vi "SW_Prepare_Conditions_Array_for_Saving.vi"(3 "Conditions presets array in":T2 {"Response"."TTL pulse length, ms" min=0.0 max=10000.0 step=10.0 format="%0.0g"; "Specifier(s)"."Validity criteria(s)"."Validity value" min=0.0 step=0.1 format="%.2g"; "Specifier(s)"."Value" step=1.0 format="%#.2g"}) -> (1 "Condition presets prepared for saving out":T1)   [LabVIEW 2018, in "Tracker.lvlib"]
uses:
  Tracker.lvlib
  Controls/CTL_Conditions_Array.ctl
  Controls/CTL_Conditions_Cluster.ctl
  Controls/CTL_Condition_type.ctl
  Controls/CTL_Comparison_type.ctl
  Controls/CTL_Validity_check_criteria.ctl
  Controls/CTL_Condition_response_type.ctl
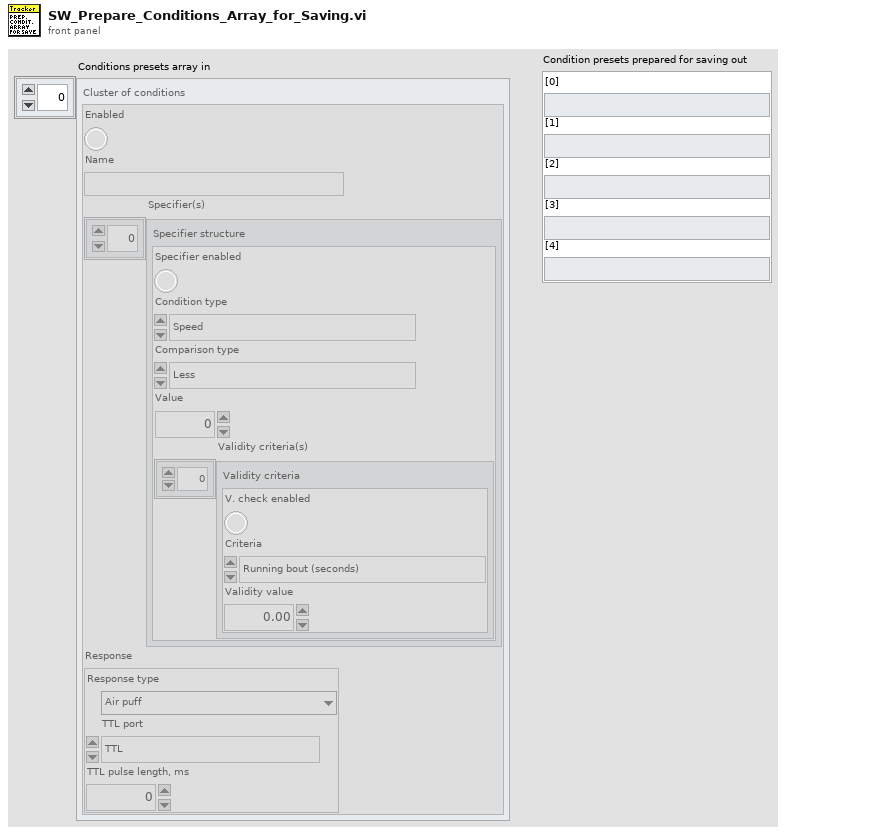
[diagram p1: front panel]
types:
  T1 = cluster{"[0]":string, "[1]":string, "[2]":string, "[3]":string, "[4]":string}
  T2 = typedef "Tracker.lvlib/CTL_Conditions_Array.ctl" = T3[]
  T3 = typedef "Tracker.lvlib/CTL_Conditions_Cluster.ctl" = cluster{"Enabled":bool, "Name":string, "Specifier(s)":cluster{"Specifier enabled":bool, "Condition type":T4, "Comparison type":T5, "Value":dbl, "Validity criteria(s)":cluster{"V. check enabled":bool, "Criteria":T6, "Validity value":dbl}[]}[], "Response":cluster{"Response type":T7, "TTL port":enum16{"TTL"}, "TTL pulse length, ms":dbl}}
  T4 = typedef "Tracker.lvlib/CTL_Condition_type.ctl" = enum16{"Speed", "Zone", "Angle to wall"}
  T5 = typedef "Tracker.lvlib/CTL_Comparison_type.ctl" = enum16{"Less", "Less or Equal", "Equal", "Greater or Equal", "Greater", "Not Equal"}
  T6 = typedef "Tracker.lvlib/CTL_Validity_check_criteria.ctl" = enum16{"Running bout (seconds)", "Running bout (meters)"}
  T7 = typedef "Tracker.lvlib/CTL_Condition_response_type.ctl" = enum16{"None", "Air puff", "Liquid reward"}
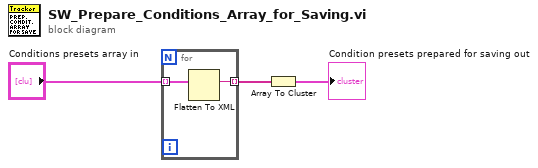
[diagram p0: block diagram]
diagram:
  n1 = for {
    tunnel: "Conditions presets array in" -> [w5] mode=indexing
    tunnel: [w4] -> w2 mode=indexing
    n2 = Flatten To XML(anything=w5) -> (xml string=w4:string)
  }
  n3 = Array To Cluster(array=w2) -> (cluster=→"Condition presets prepared for saving out":T1)
